vi "IGC100 Open Bk.vi"(3 "VISA in":refnum<visa-resource-name>="COM1") -> (0 "error out":errorcluster, 1 "VISA out":refnum<visa-resource-name>)   [LabVIEW 2010]
panel:
  in  "Pressure unit":T1(ring)
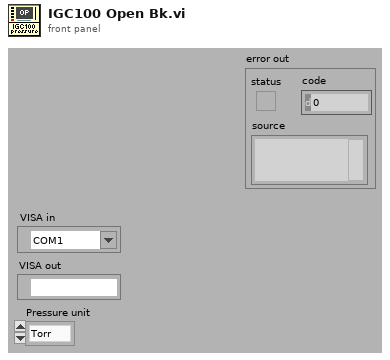
[diagram p1: front panel]
types:
  T1 = enum16{"Torr", "micron", "bar", "mbar", "Pascal"}
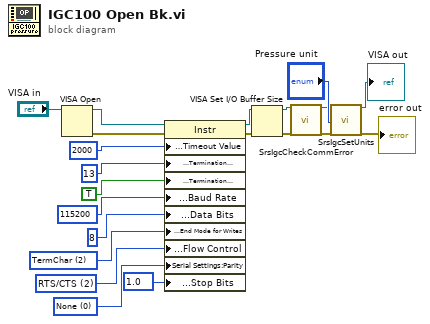
[diagram p0: block diagram]
diagram:
  w11 = u16 10 items=["1.0"=10, "1.5"=15, "2.0"=20] ("Serial Settings:Serial Stop Bits")
  w12 = u16 0 items=["None", "Odd", "Even", "Mark", "Space"] ("Serial Settings:Serial Parity")
  w13 = u16 2 items=["None"=0, "XON/XOFF"=1, "RTS/CTS"=2, "DTR/DSR"=4] ("Serial Settings:Serial Flow Control")
  w14 = u16 2 items=["None", "LastBit", "TermChar", "Break"] ("Serial Settings:Serial End Mode for Writes")
  n1 = VISA Open(VISA resource name="VISA in") -> (VISA resource name=w7:refnum<visa-resource-name>, error out=w8:errorcluster)  [unwired: 4 in]
  n2 = property class="Instr"(reference=w7, error in=w8, "General Settings:Timeout Value"=u32 2000, "Message Based Settings:Termination Character"=u8 13, "Message Based Settings:Termination Character Enable"=TRUE, "Serial Settings:Baud Rate"=u32 115200 ("Serial Settings:Serial Baud Rate"), "Serial Settings:Data Bits"=u16 8 ("Serial Settings:Serial Data Bits"), "Serial Settings:End Mode for Writes"=w14, "Serial Settings:Flow Control"=w13, "Serial Settings:Parity"=w12, "Serial Settings:Stop Bits"=w11) -> (reference out=w10:refnum<visa-resource-name>, error out=w9:errorcluster)
  n3 = VISA Set I/O Buffer Size(VISA resource name=w10, error in (no error)=w9) -> (VISA resource name out=w6:refnum<visa-resource-name>, error out=w5:errorcluster)  [unwired: 2 in]
  n4 = call "SrsIgcCheckCommError.vi"("VISA in"=w6, "error in"=w5) -> ("VISA out"=w4:refnum<visa-resource-name>, "error out"=w2:errorcluster)  [unwired: 16 in]
  n5 = call "SrsIgcSetUnits.vi"("VISA in"=w4, "Units In"="Pressure unit", "Error In"=w2) -> ("VISA out"=→"VISA out":refnum<visa-resource-name>, "error out"=→"error out":errorcluster)  [unwired: 14 in, 1 out]
